vi "BoundAngleNeg180to180.vi"(1 "angle":dbl) -> (0 "bound angle":dbl)   [LabVIEW 2015]
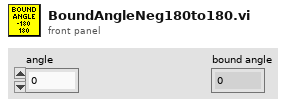
[diagram p1: front panel]
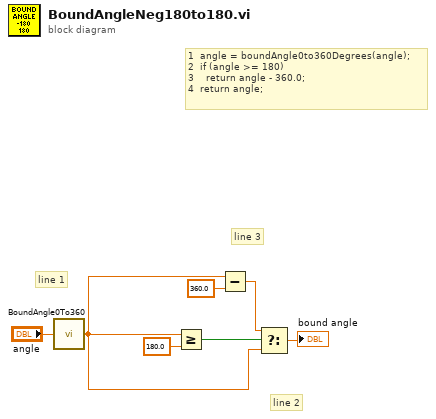
[diagram p0: block diagram]
diagram:
  # "line 1"
  # "line 3"
  # "1  angle = boundAngle0to360Degrees(angle);\n2  if (angle >= 180)\n3    return angle - 360.0;\n4  return angle;"
  # "line 2"
  n1 = call "BoundAngle0To360.vi"("angle"="angle") -> ("bound angle"=w2:dbl)
  n2 = Greater Or Equal?(x=w2, y=180.0) -> (x >= y?=w5:bool)
  n3 = Subtract(x=w2, y=360.0) -> (x-y=w4:dbl)
  n4 = Select(t=w4, s=w5, f=w2) -> (s? t:f=→"bound angle":dbl)
